vi "2_1.vi"() -> ()   [LabVIEW 2021]
panel:
  out "x*y":i32
  out "Vertical (depth)":i32
  out "Horizontal":i32
  out "Formatted 1D String Array":string[](array[string])
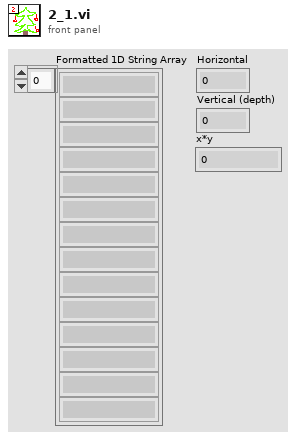
[diagram p1: front panel]
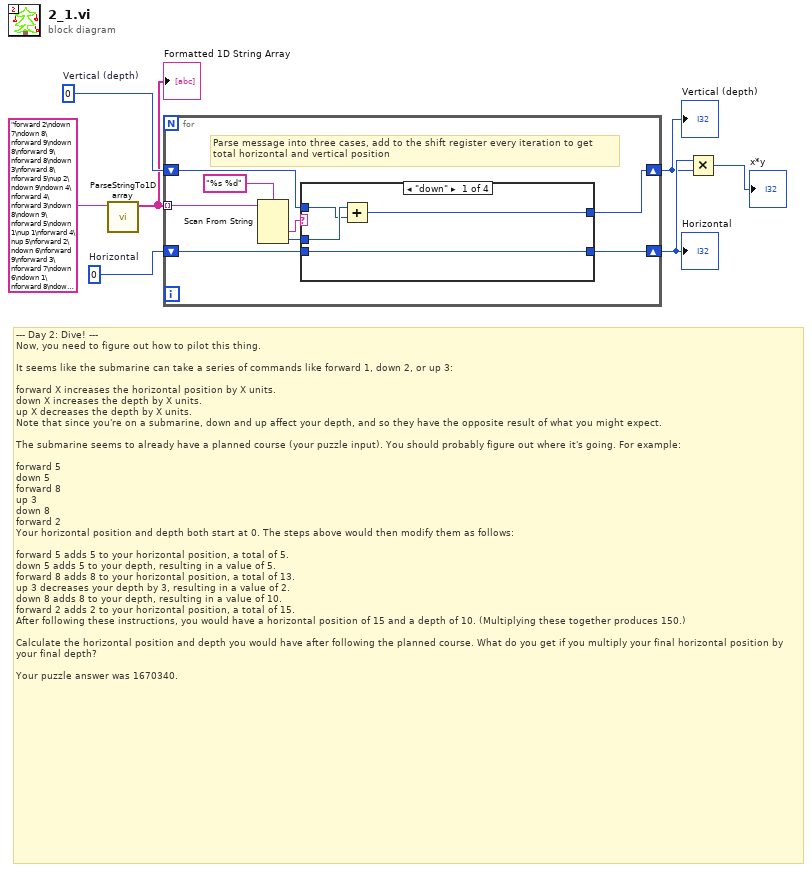
[diagram p0: block diagram]
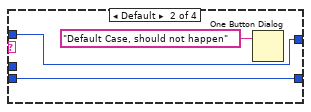
[diagram p2: hidden frame]
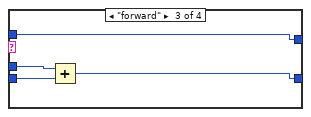
[diagram p3: hidden frame]
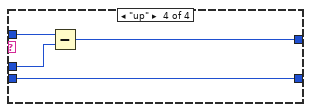
[diagram p4: hidden frame]
diagram:
  w6 = 0  # Vertical (depth)
  w7 = 0  # Horizontal
  # "--- Day 2: Dive! ---\nNow, you need to figure out how to pilot this thing.\n\nIt seems like the submarine can take a series of commands like forward 1, down 2, or up 3:\n\nforward X increases the horizontal position by X units.\ndown X increases the depth by X units.\nup X decreases the depth by X units.\nNote that since you're on a submarine, down and up affect your depth, and so they have the opposite result of what you might expect.\n\nThe submarine seems to already have a planned course (your puzzle input). You should probably figure out where it's going. For example:\n\nforward 5\ndown 5\nforward 8\nup 3\ndown 8\nforward 2\nYour horizontal position and depth both start at 0. The steps above would then modify them as follows:\n\nforward 5 adds 5 to your horizontal position, a total of 5.\ndown 5 adds 5 to your depth, resulting in a value of 5.\nforward 8 adds 8 to your horizontal position, a total of 13.\nup 3 decreases your depth by 3, resulting in a value of 2.\ndown 8 adds 8 to your depth, resulting in a value of 10.\nforward 2 adds 2 to your horizontal position, a total of 15.\nAfter following these instructions, you would have a horizontal position of 15 and a depth of 10. (Multiplying these together produces 150.)\n\nCalculate the horizontal position and depth you would have after following the planned course. What do you get if you multiply your final horizontal position by your final depth?\n\nYour puzzle answer was 1670340."
  n1 = call "ParseStringTo1Darray.vi"("Copied Input From Advent Of Code Website"="forward 2\ndown 7\ndown 8\nforward 9\ndown 8\nforward 9\nforward 8\ndown 3\nforward 8\nforward 5\nup 2\ndown 9\ndown 4\nforward 4\nforward 3\ndown 8\ndown 9\nforward 5\ndown 1\nup 1\nforward 4\nup 5\nforward 2\ndown 6\nforward 9\nforward 3\nforward 7\ndown 6\ndown 1\nforward 8\ndown 3\nforward 1\nup 6\ndown 1\ndown 2\nforward 9\ndown 7\ndown 1\ndown 7\ndown 7\nup 5\ndown 8\nforward 6\nup 8\nup 2\nforward 6\nup 1\ndown 9\nforward 8\nforward 4\nup 3\nforward 7\ndown 2\ndown 8\nforward 5\ndown 9\nup 4\nforward 7\nforward 5\ndown 5\ndown 5\nforward 3\nforward 2\ndown 2\nup 4\nup 7\ndown 8\nup 8\nforward 1\nup 4\nforward 4\ndown 2\nforward 5\nforward 7\ndown 4\nforward 8\ndown 2\nforward 5\nforward 9\nforward 6\nforward 5\ndown 5\nforward 4\nforward 3\ndown 7\ndown 8\nforward 9\nforward 7\ndown 3\ndown 6\nforward 4\ndown 7\nup 9\ndown 8\nup 7\nup 3\nforward 6\nforward 9\ndown 2\ndown 3\ndown 1\ndown 3\nforward 8\nforward 3\nforward 9\ndown 5\nup 1\nup 2\ndown 9\nup 9\ndown 5\ndown 9\nforward 1\ndown 3\ndown 5\ndown 1\nforward 7\ndown 6\nforward 7\nforward 4\nup 2\nup 1\nforward 9\ndown 2\ndown 6\ndown 5\ndown 6\nforward 8\ndown 5\nforward 1\nforward 2\ndown 7\ndown 5\ndown 7\nup 9\ndown 9\nup 4\ndown 7\nup 8\ndown 9\nforward 3\ndown 6\ndown 2\nforward 9\ndown 4\nup 7\nforward 3\ndown 5\nforward 8\nforward 9\ndown 2\nup 5\nforward 2\nforward 9\nup 5\ndown 2\nforward 8\nforward 6\ndown 7\ndown 3\nforward 4\nforward 3\nforward 9\nup 4\nup 4\nforward 7\nup 3\nforward 6\ndown 7\nup 8\nforward 2\nup 1\ndown 6\nforward 4\nup 6\nup 6\nup 3\nforward 4\nforward 2\nforward 5\nforward 8\ndown 9\ndown 4\ndown 3\ndown 1\ndown 6\ndown 4\ndown 5\ndown 7\ndown 5\nup 4\nforward 3\ndown 4\ndown 7\ndown 7\ndown 2\nforward 2\nforward 9\nup 6\ndown 3\nup 9\nforward 8\ndown 9\nup 2\nup 2\nup 2\nup 1\ndown 6\nforward 9\nforward 2\nforward 2\nforward 2\nforward 5\nup 3\ndown 7\ndown 6\ndown 8\nup 3\nup 9\ndown 3\nforward 1\nforward 7\ndown 7\ndown 1\nforward 3\ndown 7\ndown 9\ndown 7\ndown 3\nup 2\ndown 6\nup 6\ndown 1\nup 2\nforward 7\nup 2\ndown 7\nup 2\ndown 9\ndown 3\nforward 6\ndown 5\ndown 1\nforward 5\ndown 2\ndown 6\ndown 1\ndown 3\ndown 3\ndown 5\nforward 2\nforward 4\nforward 8\nforward 6\nforward 4\nforward 9\nup 8\ndown 5\nforward 1\ndown 1\nforward 1\nforward 6\nup 1\ndown 6\ndown 3\nforward 9\nforward 5\nforward 4\nup 3\nup 7\ndown 2\nup 4\nup 2\ndown 1\nforward 6\nforward 9\nforward 4\nforward 2\ndown 8\nforward 4\nforward 3\nup 5\ndown 4\nforward 3\ndown 8\ndown 5\ndown 5\nforward 1\nforward 6\nforward 4\nforward 5\nforward 9\nforward 5\ndown 4\nforward 3\nforward 8\ndown 8\ndown 1\nup 4\ndown 4\nup 7\nforward 2\nforward 6\ndown 3\ndown 5\ndown 5\ndown 8\nup 3\ndown 2\nforward 4\nforward 2\nforward 4\nforward 9\nup 2\ndown 7\nup 7\ndown 2\nforward 4\nup 7\nforward 4\ndown 2\nforward 7\nup 2\ndown 3\nforward 5\ndown 7\ndown 2\nup 2\nup 1\nup 7\nup 9\ndown 3\nforward 1\nforward 3\ndown 2\ndown 3\nforward 6\ndown 7\nforward 9\ndown 9\nforward 3\nforward 2\ndown 1\nup 9\ndown 4\nforward 4\nup 4\nforward 7\nup 3\ndown 4\ndown 9\ndown 3\nforward 7\ndown 6\ndown 7\ndown 6\nup 5\nforward 3\nforward 9\nup 2\nup 4\nup 9\ndown 2\nforward 5\nup 1\ndown 7\ndown 5\nup 2\nforward 8\ndown 8\nup 3\nforward 4\ndown 9\nforward 6\ndown 9\ndown 5\nforward 6\ndown 8\nup 6\ndown 3\nforward 6\nforward 3\ndown 3\ndown 5\ndown 7\ndown 1\ndown 5\ndown 7\ndown 5\nforward 3\ndown 2\nforward 4\nup 4\nup 1\nup 7\nforward 1\nforward 5\ndown 4\ndown 8\ndown 3\nforward 4\ndown 3\nup 7\ndown 6\nforward 9\nup 8\nforward 2\nforward 5\ndown 6\nup 4\nforward 8\nforward 5\ndown 6\nforward 2\ndown 7\nforward 3\nforward 1\nforward 6\ndown 9\nup 6\ndown 4\ndown 2\nup 8\nforward 4\ndown 8\nforward 8\nup 9\nforward 7\ndown 6\nup 9\ndown 4\nup 6\ndown 4\ndown 3\nup 7\nup 4\nforward 5\nup 9\ndown 9\nup 6\ndown 3\nforward 8\ndown 9\nforward 7\nup 3\nup 9\nforward 8\ndown 3\nforward 3\nforward 5\ndown 6\nforward 3\ndown 4\nup 6\nforward 3\nforward 7\ndown 1\ndown 6\ndown 4\nforward 6\nup 6\ndown 5\ndown 6\ndown 4\nup 2\ndown 7\ndown 9\ndown 2\ndown 6\nforward 3\nforward 4\ndown 5\nup 5\ndown 5\nforward 3\nforward 6\ndown 4\ndown 7\nup 2\nforward 7\ndown 7\nup 6\nup 3\nforward 9\nforward 8\nup 6\nforward 2\ndown 2\nforward 8\nforward 4\nup 6\nforward 6\ndown 8\nup 3\nup 5\nforward 6\nup 8\ndown 1\ndown 4\nup 9\nforward 6\nup 5\ndown 6\ndown 8\ndown 9\nforward 5\nup 3\ndown 7\nforward 3\nforward 6\ndown 3\ndown 1\ndown 9\nup 9\ndown 4\ndown 7\nforward 2\nforward 4\ndown 7\nforward 7\nup 5\ndown 9\nup 7\ndown 4\nforward 6\ndown 5\nforward 4\nup 8\ndown 4\ndown 7\nforward 3\ndown 6\ndown 1\nforward 3\ndown 4\nup 6\nup 5\nup 7\nforward 5\ndown 4\nforward 7\nup 1\ndown 4\nforward 4\ndown 2\ndown 6\nforward 1\nup 3\nup 8\nforward 6\nforward 6\ndown 5\nforward 7\ndown 6\ndown 8\nforward 6\ndown 6\nforward 3\nforward 5\ndown 9\ndown 5\nup 4\ndown 5\ndown 1\nforward 1\nforward 5\ndown 2\nforward 5\nforward 2\nforward 5\nup 3\nforward 5\nup 8\nforward 9\nforward 3\ndown 2\nup 2\nforward 7\ndown 5\nup 1\ndown 3\ndown 7\nup 2\nforward 8\nforward 6\nforward 1\nforward 6\nforward 6\ndown 5\nforward 4\ndown 5\nforward 9\nforward 7\ndown 7\ndown 7\ndown 9\nforward 4\ndown 4\nforward 3\ndown 6\nforward 5\ndown 9\nforward 6\nup 7\ndown 3\nup 4\nup 4\ndown 1\ndown 2\nup 5\nforward 6\nforward 2\ndown 7\nup 6\nup 3\ndown 8\nforward 1\ndown 3\nup 9\ndown 2\nforward 6\nforward 1\nforward 4\nup 1\ndown 8\ndown 2\ndown 9\ndown 5\nforward 3\ndown 1\ndown 6\ndown 5\ndown 3\nforward 1\nforward 9\nup 2\ndown 3\ndown 3\ndown 9\ndown 7\nforward 6\nforward 8\nforward 4\nup 7\ndown 2\nforward 3\nforward 1\nup 4\nforward 8\nup 9\nforward 8\nforward 2\ndown 5\nforward 2\ndown 6\ndown 6\ndown 4\nforward 8\ndown 6\nforward 2\nforward 8\ndown 7\ndown 6\nforward 2\ndown 1\ndown 8\nforward 2\nforward 9\nup 6\nforward 6\ndown 3\ndown 2\nup 5\nup 6\ndown 6\nup 7\nforward 5\nforward 7\ndown 1\nforward 7\nforward 9\ndown 3\nforward 4\nforward 5\ndown 1\nup 3\nforward 2\nup 5\nforward 2\nforward 1\ndown 5\ndown 4\ndown 8\nup 8\nforward 3\ndown 3\nforward 4\ndown 6\nup 8\ndown 5\nup 2\ndown 1\nup 3\nforward 8\nup 6\nforward 9\nup 9\ndown 5\nforward 2\nforward 9\nup 6\nforward 1\ndown 2\nforward 4\nforward 4\nforward 1\nforward 5\nforward 1\nforward 4\ndown 5\ndown 1\ndown 2\ndown 2\nforward 7\ndown 7\ndown 7\ndown 4\ndown 7\ndown 4\ndown 3\nup 7\nup 1\nforward 2\nforward 3\ndown 4\ndown 5\nforward 9\nup 7\nforward 6\ndown 1\nforward 6\nforward 6\nforward 8\ndown 3\nforward 2\ndown 6\nforward 9\nup 6\nup 6\nforward 7\ndown 5\ndown 6\nup 3\ndown 5\nup 4\nforward 3\ndown 7\nforward 9\nup 1\ndown 1\nup 6\ndown 3\nup 2\ndown 5\nforward 3\nforward 6\ndown 9\ndown 4\nforward 7\ndown 1\nup 1\nforward 3\nforward 5\nup 7\ndown 3\nup 9\nup 9\ndown 4\nup 4\nforward 8\nup 9\ndown 8\nforward 6\nforward 4\nforward 9\nforward 8\ndown 2\nforward 3\nforward 2\ndown 3\nup 1\nforward 6\ndown 3\ndown 7\ndown 3\ndown 5\ndown 9\nup 9\nforward 8\nforward 6\ndown 8\nforward 3\ndown 4\ndown 2\ndown 9\nforward 4\nforward 2\nup 4\nforward 1\nup 8\nup 1\ndown 4\nup 2\ndown 1\nup 7\ndown 2\ndown 4\nup 4\nforward 2\ndown 3\nforward 2\nforward 3\ndown 5\nforward 9\nforward 7\ndown 1\nup 3\ndown 3\nforward 3\ndown 6\nforward 5\nup 3\nup 3\nup 1\nforward 7\nforward 1\nforward 2\nforward 2\ndown 4\nup 7\nforward 1\nforward 1\nforward 6\ndown 8\nup 8\ndown 8\ndown 4\ndown 6\nforward 8\nforward 4\nforward 5\ndown 2\ndown 3\nforward 7\ndown 6\nforward 4\nforward 1\nup 7\nup 5\nup 2\nforward 1\nforward 8\nforward 2\nup 9\nforward 4\nforward 5\ndown 2\nforward 5\nforward 7\ndown 3\nforward 1\ndown 3\nup 5\nup 2\nup 2\nup 2\nforward 4\nforward 4\nforward 8\nforward 2\ndown 3\nup 7\ndown 4\ndown 2\ndown 7\nforward 2\ndown 2\nforward 7\nup 9\nup 7\nforward 7\nforward 7\ndown 3\ndown 4\nup 4\ndown 2\ndown 8\nforward 4\ndown 1\nup 6\nforward 4\ndown 2\nup 8\ndown 1\ndown 8\ndown 6\nup 9\nforward 4\nup 1\ndown 2\ndown 9\ndown 7\ndown 4\ndown 8\ndown 8\nup 1\ndown 5\nup 5\ndown 7\nup 7\nforward 5\ndown 3\nforward 7\nup 5\ndown 3\nforward 9\nup 5\ndown 7\nforward 8\nforward 8\ndown 2\nforward 7\nforward 8\ndown 4\nup 7\ndown 2\nup 7\nforward 5\ndown 1\ndown 3\nforward 9\nup 4\nforward 6\nforward 4\ndown 5\ndown 7\nforward 2\nforward 4\ndown 2\nforward 1\ndown 5\nup 2\ndown 8\ndown 1\ndown 4\ndown 8\ndown 6\nforward 9\nforward 2\nforward 6\nforward 4\ndown 1\nforward 8\nup 4\nforward 6\ndown 4\nforward 4\nforward 3\nforward 6\nforward 9\nforward 8\ndown 1\nforward 5\ndown 8\nforward 7\nup 1\ndown 3\nup 6\nforward 5\nforward 8\nforward 8\nforward 5\nforward 5\nforward 1\nup 9\nforward 7\nup 3\ndown 2\ndown 4\nforward 6\nup 2\nforward 5\nup 8\nforward 8\nforward 2\nforward 6\nforward 3\nup 4\nforward 3\nforward 6" ("String")) -> ("Formatted 1D String Array"=w4:string[])  [unwired: 10 in]
  "Formatted 1D String Array" <- w4
  n2 = for {
    shift-right: [w9] -> w2
    shift-left: w6 -> [w10]
    shift-right: [w11] -> w3
    shift-left: w7 -> [w12]
    tunnel: w4 -> [w15] mode=indexing
    # "Parse message into three cases, add to the shift register every iteration to get \ntotal horizontal and vertical position"
    n3 = Scan From String(format string="%s %d", input string=w15) -> (output 1=w13:string, output 2=w8:i32)  [unwired: 4 in, 3 out]
    n4 = case shown="\"down\"" w13 {
      tunnel: w12 -> [w19 w22 w24 w30]
      tunnel: [w19 w22 w23 w30] -> w11
      tunnel: w10 -> [w17 w21 w26 w29]
      tunnel: [w16 w21 w26 w27] -> w9
      tunnel: w8 -> [w18 _ w25 w28]
      frame "down" {
        n5 = Add(x=w18, y=w17) -> (x+y=w16:i32)
      }
      frame Default {
        n6 = One Button Dialog(message="Default Case, should not happen") -> ()  [unwired: 1 in, 1 out]
      }
      frame "forward" {
        n7 = Add(x=w25, y=w24) -> (x+y=w23:i32)
      }
      frame "up" {
        n8 = Subtract(x=w29, y=w28) -> (x-y=w27:i32)
      }
    }
  }
  "Horizontal" <- w3
  "Vertical (depth)" <- w2
  n9 = Multiply(x=w3, y=w2) -> (x*y=→"x*y":i32)
